vi "Spreadsheet Example.vi"() -> ()   [LabVIEW 2010]
doc: "This VI is an exercise in the LabVIEW Core I course.\n\nThis VI generates three data arrays, combines them into a 2D array, graphs them, and writes the 2D array of data to a file in spreadsheet format using the high-level file I/O function named Write To Spreadsheet File.vi."
uses:
  <vilib>/Utility/file.llb/Write To Spreadsheet File (DBL).vi
  <vilib>/Analysis/NI_AALBase.lvlib
panel:
  out "Waveform Graph":dbl[][](graph)
  out "Table":string[][](table)
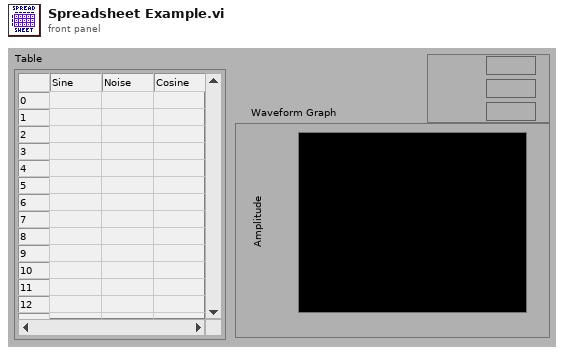
[diagram p1: front panel]
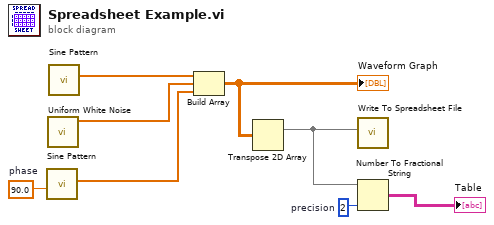
[diagram p0: block diagram]
diagram:
  w5 = 2  # precision
  w6 = 90.0  # phase
  n1 = call <vilib>:"Sine Pattern.vi"("phase(degrees)"=w6) -> ("Sinusoidal Pattern"=w1:dbl[])  [unwired: 3 in, 1 out]
  n2 = call <vilib>:"Uniform White Noise.vi"() -> ("uniform white noise"=w8:dbl[])  [unwired: 10 in, 1 out]
  n3 = call <vilib>:"Sine Pattern.vi"() -> ("Sinusoidal Pattern"=w7:dbl[])  [unwired: 4 in, 1 out]
  n4 = Build Array "Build Array"(w7, w8, w1) -> (w2:dbl[][])
  "Waveform Graph" <- w2
  n5 = Transpose 2D Array(2D array=w2) -> (transposed array=w4:dbl[][])
  n6 = call-poly <vilib>:"Write To Spreadsheet File.vi"("2D data"=w4) -> ()  [unwired: 7 in, 1 out]
  n7 = Number To Fractional String(number=w4, precision (6)=w5) -> (F-format string=→"Table":string[][])  [unwired: 2 in]
